vi "const_cluster_firesetting.vi"() -> (0 "firesetting {}":T1)   [LabVIEW 2009]
uses:
  ctl firesetting.ctl
panel:
  # "12"
  # "12"
  # "12"
  # "12``"
  # "14"
  # "12"
  # "10\n\n\n10\n\n\n10\n\n10"
  # "46"
  # "23"
  # "10"
  # "23"
  # "4"
  # "23"
  # "4"
  # "23"
  # "4"
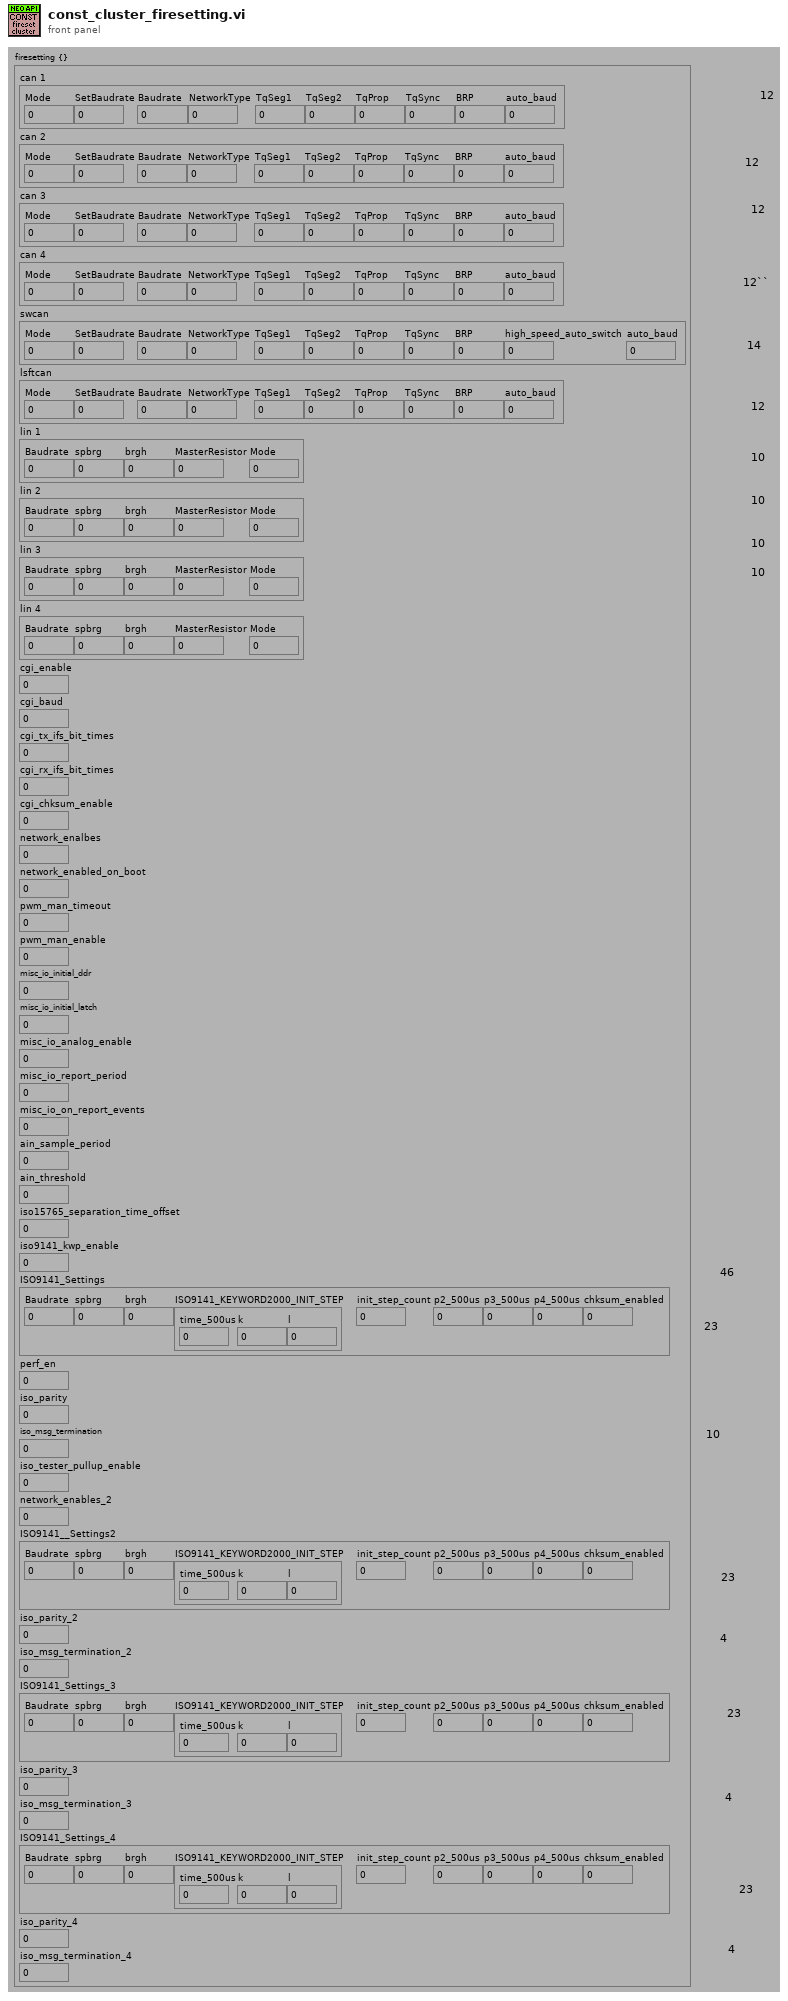
[diagram p1: front panel]
types:
  T1 = cluster{"can 1":cluster{"Mode":u8, "SetBaudrate":u8, "Baudrate":u8, "NetworkType":u8, "TqSeg1":u8, "TqSeg2":u8, "TqProp":u8, "TqSync":u8, "BRP":u16, "auto_baud":u16}, "can 2":cluster{"Mode":u8, "SetBaudrate":u8, "Baudrate":u8, "NetworkType":u8, "TqSeg1":u8, "TqSeg2":u8, "TqProp":u8, "TqSync":u8, "BRP":u16, "auto_baud":u16}, "can 3":cluster{"Mode":u8, "SetBaudrate":u8, "Baudrate":u8, "NetworkType":u8, "TqSeg1":u8, "TqSeg2":u8, "TqProp":u8, "TqSync":u8, "BRP":u16, "auto_baud":u16}, "can 4":cluster{"Mode":u8, "SetBaudrate":u8, "Baudrate":u8, "NetworkType":u8, "TqSeg1":u8, "TqSeg2":u8, "TqProp":u8, "TqSync":u8, "BRP":u16, "auto_baud":u16}, "swcan":cluster{"Mode":u8, "SetBaudrate":u8, "Baudrate":u8, "NetworkType":u8, "TqSeg1":u8, "TqSeg2":u8, "TqProp":u8, "TqSync":u8, "BRP":u16, "high_speed_auto_switch":u16, "auto_baud":u16}, "lsftcan":cluster{"Mode":u8, "SetBaudrate":u8, "Baudrate":u8, "NetworkType":u8, "TqSeg1":u8, "TqSeg2":u8, "TqProp":u8, "TqSync":u8, "BRP":u16, "auto_baud":u16}, "lin 1":cluster{"Baudrate":u32, "spbrg":u16, "brgh":u16, "MasterResistor":u8, "Mode":u8}, "lin 2":cluster{"Baudrate":u32, "spbrg":u16, "brgh":u16, "MasterResistor":u8, "Mode":u8}, "lin 3":cluster{"Baudrate":u32, "spbrg":u16, "brgh":u16, "MasterResistor":u8, "Mode":u8}, "lin 4":cluster{"Baudrate":u32, "spbrg":u16, "brgh":u16, "MasterResistor":u8, "Mode":u8}, "cgi_enable":u16, "cgi_baud":u16, "cgi_tx_ifs_bit_times":u16, "cgi_rx_ifs_bit_times":u16, "cgi_chksum_enable":u16, "network_enalbes":u16, "network_enabled_on_boot":u16, "pwm_man_timeout":u16, "pwm_man_enable":u16, "misc_io_initial_ddr":u16, "misc_io_initial_latch":u16, "misc_io_analog_enable":u16, "misc_io_report_period":u16, "misc_io_on_report_events":u16, "ain_sample_period":u16, "ain_threshold":u16, "iso15765_separation_time_offset":u16, "iso9141_kwp_enable":u16, "ISO9141_Settings":cluster{"Baudrate":u32, "spbrg":u16, "brgh":u16, "ISO9141_KEYWORD2000_INIT_STEP":cluster{"time_500us":u16, "k":u16, "l":u16}, "init_step_count":u8, "p2_500us":u16, "p3_500us":u16, "p4_500us":u16, "chksum_enabled":u16}, "perf_en":u16, "iso_parity":u16, "iso_msg_termination":u16, "iso_tester_pullup_enable":u16, "network_enables_2":u16, "ISO9141__Settings2":cluster{"Baudrate":u32, "spbrg":u16, "brgh":u16, "ISO9141_KEYWORD2000_INIT_STEP":cluster{"time_500us":u16, "k":u16, "l":u16}, "init_step_count":u8, "p2_500us":u16, "p3_500us":u16, "p4_500us":u16, "chksum_enabled":u16}, "iso_parity_2":u16, "iso_msg_termination_2":u16, "ISO9141_Settings_3":cluster{"Baudrate":u32, "spbrg":u16, "brgh":u16, "ISO9141_KEYWORD2000_INIT_STEP":cluster{"time_500us":u16, "k":u16, "l":u16}, "init_step_count":u8, "p2_500us":u16, "p3_500us":u16, "p4_500us":u16, "chksum_enabled":u16}, "iso_parity_3":u16, "iso_msg_termination_3":u16, "ISO9141_Settings_4":cluster{"Baudrate":u32, "spbrg":u16, "brgh":u16, "ISO9141_KEYWORD2000_INIT_STEP":cluster{"time_500us":u16, "k":u16, "l":u16}, "init_step_count":u8, "p2_500us":u16, "p3_500us":u16, "p4_500us":u16, "chksum_enabled":u16}, "iso_parity_4":u16, "iso_msg_termination_4":u16}
  T2 = typedef "ctl FireSetting.ctl" = cluster{"can 1":cluster{"Mode":u8, "SetBaudrate":u8, "Baudrate":u8, "NetworkType":u8, "TqSeg1":u8, "TqSeg2":u8, "TqProp":u8, "TqSync":u8, "BRP":u16, "auto_baud":u16}, "can 2":cluster{"Mode":u8, "SetBaudrate":u8, "Baudrate":u8, "NetworkType":u8, "TqSeg1":u8, "TqSeg2":u8, "TqProp":u8, "TqSync":u8, "BRP":u16, "auto_baud":u16}, "can 3":cluster{"Mode":u8, "SetBaudrate":u8, "Baudrate":u8, "NetworkType":u8, "TqSeg1":u8, "TqSeg2":u8, "TqProp":u8, "TqSync":u8, "BRP":u16, "auto_baud":u16}, "can 4":cluster{"Mode":u8, "SetBaudrate":u8, "Baudrate":u8, "NetworkType":u8, "TqSeg1":u8, "TqSeg2":u8, "TqProp":u8, "TqSync":u8, "BRP":u16, "auto_baud":u16}, "swcan":cluster{"Mode":u8, "SetBaudrate":u8, "Baudrate":u8, "NetworkType":u8, "TqSeg1":u8, "TqSeg2":u8, "TqProp":u8, "TqSync":u8, "BRP":u16, "high_speed_auto_switch":u16, "auto_baud":u16}, "lsftcan":cluster{"Mode":u8, "SetBaudrate":u8, "Baudrate":u8, "NetworkType":u8, "TqSeg1":u8, "TqSeg2":u8, "TqProp":u8, "TqSync":u8, "BRP":u16, "auto_baud":u16}, "lin 1":cluster{"Baudrate":u32, "spbrg":u16, "brgh":u16, "MasterResistor":u8, "Mode":u8}, "lin 2":cluster{"Baudrate":u32, "spbrg":u16, "brgh":u16, "MasterResistor":u8, "Mode":u8}, "lin 3":cluster{"Baudrate":u32, "spbrg":u16, "brgh":u16, "MasterResistor":u8, "Mode":u8}, "lin 4":cluster{"Baudrate":u32, "spbrg":u16, "brgh":u16, "MasterResistor":u8, "Mode":u8}, "cgi_enable":u16, "cgi_baud":u16, "cgi_tx_ifs_bit_times":u16, "cgi_rx_ifs_bit_times":u16, "cgi_chksum_enable":u16, "network_enalbes":u16, "network_enabled_on_boot":u16, "pwm_man_timeout":u16, "pwm_man_enable":u16, "misc_io_initial_ddr":u16, "misc_io_initial_latch":u16, "misc_io_analog_enable":u16, "misc_io_report_period":u16, "misc_io_on_report_events":u16, "ain_sample_period":u16, "ain_threshold":u16, "iso15765_separation_time_offset":u16, "iso9141_kwp_enable":u16, "ISO9141_Settings":cluster{"Baudrate":u32, "spbrg":u16, "brgh":u16, "ISO9141_KEYWORD2000_INIT_STEP":cluster{"time_500us":u16, "k":u16, "l":u16}, "init_step_count":u8, "p2_500us":u16, "p3_500us":u16, "p4_500us":u16, "chksum_enabled":u16}, "perf_en":u16, "iso_parity":u16, "iso_msg_termination":u16, "iso_tester_pullup_enable":u16, "network_enables_2":u16, "ISO9141__Settings2":cluster{"Baudrate":u32, "spbrg":u16, "brgh":u16, "ISO9141_KEYWORD2000_INIT_STEP":cluster{"time_500us":u16, "k":u16, "l":u16}, "init_step_count":u8, "p2_500us":u16, "p3_500us":u16, "p4_500us":u16, "chksum_enabled":u16}, "iso_parity_2":u16, "iso_msg_termination_2":u16, "ISO9141_Settings_3":cluster{"Baudrate":u32, "spbrg":u16, "brgh":u16, "ISO9141_KEYWORD2000_INIT_STEP":cluster{"time_500us":u16, "k":u16, "l":u16}, "init_step_count":u8, "p2_500us":u16, "p3_500us":u16, "p4_500us":u16, "chksum_enabled":u16}, "iso_parity_3":u16, "iso_msg_termination_3":u16, "ISO9141_Settings_4":cluster{"Baudrate":u32, "spbrg":u16, "brgh":u16, "ISO9141_KEYWORD2000_INIT_STEP":cluster{"time_500us":u16, "k":u16, "l":u16}, "init_step_count":u8, "p2_500us":u16, "p3_500us":u16, "p4_500us":u16, "chksum_enabled":u16}, "iso_parity_4":u16, "iso_msg_termination_4":u16}
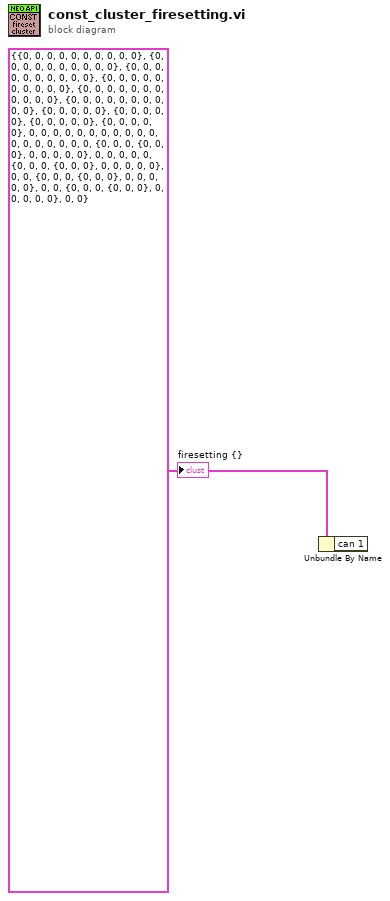
[diagram p0: block diagram]
diagram:
  w1 = T2 {"can 1"={"Mode"=0, "SetBaudrate"=0, "Baudrate"=0, "NetworkType"=0, "TqSeg1"=0, "TqSeg2"=0, "TqProp"=0, "TqSync"=0, "BRP"=0, "auto_baud"=0}, "can 2"={"Mode"=0, "SetBaudrate"=0, "Baudrate"=0, "NetworkType"=0, "TqSeg1"=0, "TqSeg2"=0, "TqProp"=0, "TqSync"=0, "BRP"=0, "auto_baud"=0}, "can 3"={"Mode"=0, "SetBaudrate"=0, "Baudrate"=0, "NetworkType"=0, "TqSeg1"=0, "TqSeg2"=0, "TqProp"=0, "TqSync"=0, "BRP"=0, "auto_baud"=0}, "can 4"={"Mode"=0, "SetBaudrate"=0, "Baudrate"=0, "NetworkType"=0, "TqSeg1"=0, "TqSeg2"=0, "TqProp"=0, "TqSync"=0, "BRP"=0, "auto_baud"=0}, "swcan"={"Mode"=0, "SetBaudrate"=0, "Baudrate"=0, "NetworkType"=0, "TqSeg1"=0, "TqSeg2"=0, "TqProp"=0, "TqSync"=0, "BRP"=0, "high_speed_auto_switch"=0, "auto_baud"=0}, "lsftcan"={"Mode"=0, "SetBaudrate"=0, "Baudrate"=0, "NetworkType"=0, "TqSeg1"=0, "TqSeg2"=0, "TqProp"=0, "TqSync"=0, "BRP"=0, "auto_baud"=0}, "lin 1"={"Baudrate"=0, "spbrg"=0, "brgh"=0, "MasterResistor"=0, "Mode"=0}, "lin 2"={"Baudrate"=0, "spbrg"=0, "brgh"=0, "MasterResistor"=0, "Mode"=0}, "lin 3"={"Baudrate"=0, "spbrg"=0, "brgh"=0, "MasterResistor"=0, "Mode"=0}, "lin 4"={"Baudrate"=0, "spbrg"=0, "brgh"=0, "MasterResistor"=0, "Mode"=0}, "cgi_enable"=0, "cgi_baud"=0, "cgi_tx_ifs_bit_times"=0, "cgi_rx_ifs_bit_times"=0, "cgi_chksum_enable"=0, "network_enalbes"=0, "network_enabled_on_boot"=0, "pwm_man_timeout"=0, "pwm_man_enable"=0, "misc_io_initial_ddr"=0, "misc_io_initial_latch"=0, "misc_io_analog_enable"=0, "misc_io_report_period"=0, "misc_io_on_report_events"=0, "ain_sample_period"=0, "ain_threshold"=0, "iso15765_separation_time_offset"=0, "iso9141_kwp_enable"=0, "ISO9141_Settings"={"Baudrate"=0, "spbrg"=0, "brgh"=0, "ISO9141_KEYWORD2000_INIT_STEP"={"time_500us"=0, "k"=0, "l"=0}, "init_step_count"=0, "p2_500us"=0, "p3_500us"=0, "p4_500us"=0, "chksum_enabled"=0}, "perf_en"=0, "iso_parity"=0, "iso_msg_termination"=0, "iso_tester_pullup_enable"=0, "network_enables_2"=0, "ISO9141__Settings2"={"Baudrate"=0, "spbrg"=0, "brgh"=0, "ISO9141_KEYWORD2000_INIT_STEP"={"time_500us"=0, "k"=0, "l"=0}, "init_step_count"=0, "p2_500us"=0, "p3_500us"=0, "p4_500us"=0, "chksum_enabled"=0}, "iso_parity_2"=0, "iso_msg_termination_2"=0, "ISO9141_Settings_3"={"Baudrate"=0, "spbrg"=0, "brgh"=0, "ISO9141_KEYWORD2000_INIT_STEP"={"time_500us"=0, "k"=0, "l"=0}, "init_step_count"=0, "p2_500us"=0, "p3_500us"=0, "p4_500us"=0, "chksum_enabled"=0}, "iso_parity_3"=0, "iso_msg_termination_3"=0, "ISO9141_Settings_4"={"Baudrate"=0, "spbrg"=0, "brgh"=0, "ISO9141_KEYWORD2000_INIT_STEP"={"time_500us"=0, "k"=0, "l"=0}, "init_step_count"=0, "p2_500us"=0, "p3_500us"=0, "p4_500us"=0, "chksum_enabled"=0}, "iso_parity_4"=0, "iso_msg_termination_4"=0} ("firesetting {}")
  n1 = Unbundle By Name(w1) -> ()  [unwired: 1 out]
  "firesetting {}" <- w1
